vi "Thev-Plot Load Impedances.vi"(2 "State":T1={"next"=-1, "ER10X"=refnum, "phase"=enum."Optimize", "progress"=[], "folder"=path "", "log"="", "history"={"L"=[], "F"=[]}, "optim"={"MSE"=0.0, "Niter"=0, "Linit"=[], "Lfinal"=[]}}, 5 "Mag graph":refnum<vi>, 7 "Phase graph":refnum<vi>, 11 "error in (no error)":errorcluster) -> (15 "error out":errorcluster)   [LabVIEW 2015]
doc: "This helper VI loads calibration data from a file, and plots the magnitude and phase on graphs whose references are inputs to the VI. Handles the logic of overplotting data, selecting the colors and linestyles, and inserting the filename into the legend.\n\nKEH 9/10/09"
uses:
  Typedefs/Thev-State.ctl
  D:/Experiment VIs/Misc VIs/Equipment Control/ER10X/ER10XConnect.NET.dll
  Misc VIs/Equipment Control/ER10X/ER10XConnect.NET.dll
  Typedefs/Thev-Procedure Phase.ctl
  Typedefs/Thev-Progress Table Element.ctl
  Typedefs/Thev-Optimization Result.ctl
  Utility VIs/Math VIs/Z to dB, degrees (1D).vi
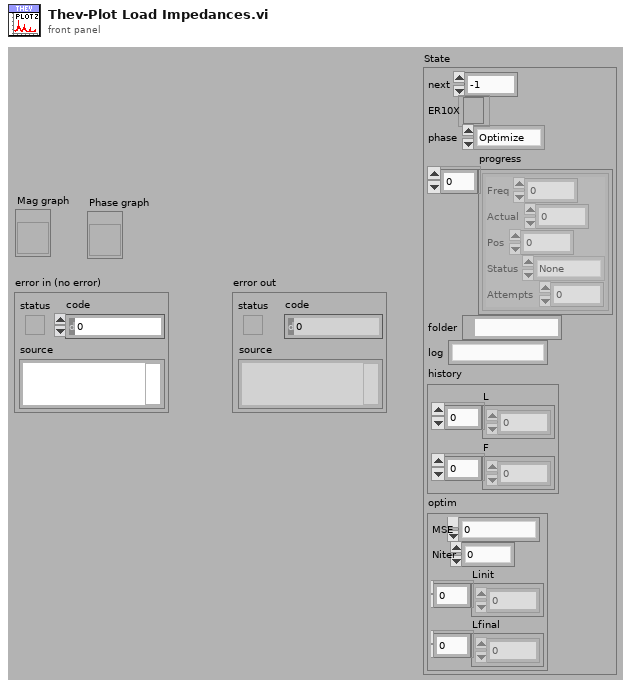
[diagram p1: front panel]
types:
  T1 = typedef "Thev-State.ctl" = cluster{"next":i32, "ER10X":refnum<k24>, "phase":T2, "progress":T3[], "folder":path, "log":string, "history":cluster{"L":dbl[], "F":dbl[]}, "optim":T4}
  T2 = typedef "Thev-Procedure Phase.ctl" = enum16{"Optimize", "Measure", "Compute", "Finished"}
  T3 = typedef "Thev-Progress Table Element.ctl" = cluster{"Freq":dbl, "Actual":dbl, "Pos":dbl, "Status":enum16{"None", "Measuring", "Finished"}, "Attempts":i32}
  T4 = typedef "Thev-Optimization Result.ctl" = cluster{"MSE":dbl, "Niter":i32, "Linit":dbl[], "Lfinal":dbl[]}
  T5 = enum16{"User", "Prism", "Kelly", "Dark2", "Sequential", "Hue"}
  T6 = cluster{"Frequency (Hz)":dbl[], "Magnitude (dB)":dbl[]}
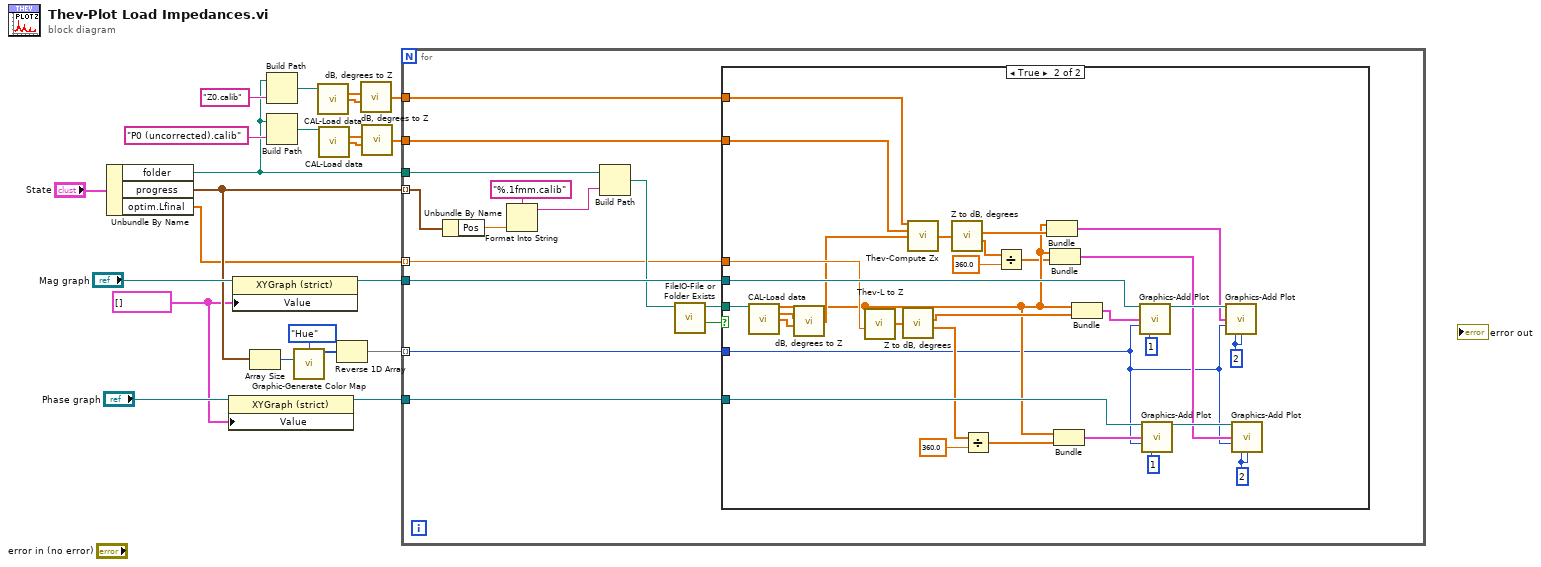
[diagram p0: block diagram]
diagram:
  w13 = cluster{"PTC Mag":dbl[], "PTC Phase":dbl[]}[] [] ("Value")
  n1 = Unbundle By Name("State") -> ("folder"=w9:path, "progress"=w18:T3[], "optim.Lfinal"=w12:dbl[])
  n2 = property class="XYGraph (strict)"(reference="Phase graph", "Value"=w13) -> (reference out=w14:refnum<vi>)  [unwired: 1 in, 1 out]
  n3 = property class="XYGraph (strict)"(reference="Mag graph", "Value"=w13) -> (reference out=w16:refnum<vi>)  [unwired: 1 in, 1 out]
  n4 = Array Size(array=w18) -> (size(s)=w19:i32)
  n5 = Build Path(base path=w9, name or relative path="Z0.calib") -> (appended path=w8:path)
  n6 = Build Path(base path=w9, name or relative path="P0 (uncorrected).calib") -> (appended path=w2:path)
  n7 = call "Graphic-Generate Color Map.vi"("Map"=T5."Hue", "Size"=w19) -> ("Colors"=w20:u32[])  [unwired: 13 in]
  n8 = call "CAL-Load data.vi"("user path"=w8) -> ("Mag"=w7:dbl[], "Phase"=w6:dbl[])  [unwired: 7 in, 6 out]
  n9 = call "CAL-Load data.vi"("user path"=w2) -> ("Mag"=w4:dbl[], "Phase"=w3:dbl[])  [unwired: 7 in, 6 out]
  n10 = Reverse 1D Array(array=w20) -> (reversed array=w17:u32[])
  n11 = call "dB, degrees to Z.vi"("Magnitude (dB)"=w7, "Phase (degrees)"=w6) -> ("Z"=w5:cdb[])  [unwired: 5 in]
  n12 = call "dB, degrees to Z.vi"("Magnitude (dB)"=w4, "Phase (degrees)"=w3) -> ("Z"=w1:cdb[])  [unwired: 5 in]
  n13 = for {
    tunnel: w16 -> [w37]
    tunnel: w9 -> [w32]
    tunnel: w18 -> [w36] mode=indexing
    tunnel: w17 -> [w31] mode=indexing
    tunnel: w14 -> [w27]
    tunnel: w12 -> [w26] mode=indexing
    tunnel: w5 -> [w25]
    tunnel: w1 -> [w24]
    n14 = Unbundle By Name(w36) -> ("Pos"=w34:dbl)
    n15 = Format Into String(format string="%.1fmm.calib", w34) -> (resulting string=w33:string)  [unwired: 2 in, 1 out]
    n16 = Build Path(base path=w32, name or relative path=w33) -> (appended path=w30:path)
    n17 = call "FileIO-File or Folder Exists.vi"("path"=w30) -> ("Exists?"=w28:bool, "dup path"=w29:path)  [unwired: 7 in, 2 out]
    n18 = case shown="True" w28 {
      tunnel: w37 -> [_ w68]
      tunnel: w31 -> [_ w38]
      tunnel: w29 -> [_ w65]
      tunnel: w27 -> [_ w61]
      tunnel: w26 -> [_ w58]
      tunnel: w25 -> [_ w53]
      tunnel: w24 -> [_ w52]
      frame False {
      }
      frame True {
        w45 = u8 2 ("Plot.Line Width")
        w46 = u8 2 ("Plot.Line Width")
        n19 = call "CAL-Load data.vi"("user path"=w65) -> ("Frequency (Hz)"=w41:dbl[], "Mag"=w60:dbl[], "Phase"=w59:dbl[])  [unwired: 7 in, 5 out]
        n20 = call "dB, degrees to Z.vi"("Magnitude (dB)"=w60, "Phase (degrees)"=w59) -> ("Z"=w51:cdb[])  [unwired: 5 in]
        n21 = call "Thev-L to Z.vi"("L (mm)"=w58, "Frequency (Hz)"=w41) -> ("Zx"=w57:cdb[])  [unwired: 2 in]
        n22 = call-poly "Z to dB, degrees.vi"("Z"=w57) -> ("Magnitude (dB)"=w56:dbl[], "Phase (degrees)"=w55:dbl[])  [unwired: 5 in]
        n23 = call "Thev-Compute Zx.vi"("Zs"=w53, "Ps"=w52, "Px"=w51) -> ("Zx"=w49:cdb[])  [unwired: 12 in]
        n24 = call-poly "Z to dB, degrees.vi"("Z"=w49) -> ("Magnitude (dB)"=w48:dbl[], "Phase (degrees)"=w43:dbl[])  [unwired: 5 in]
        n25 = Divide(x=w55, y=360.0) -> (x/y=w54:dbl[])
        n26 = Divide(x=w43, y=360.0) -> (x/y=w40:dbl[])
        n27 = Bundle("Frequency (Hz)"=w41, "Magnitude (dB)"=w48) -> (w47:T6)  [unwired: 1 in]
        n28 = Bundle("Frequency (Hz)"=w41, w40) -> (w39:cluster{"Frequency (Hz)":dbl[], dbl[]})  [unwired: 1 in]
        n29 = Bundle("Frequency (Hz)"=w41, w54) -> (w62:cluster{"Frequency (Hz)":dbl[], dbl[]})  [unwired: 1 in]
        n30 = Bundle("Frequency (Hz)"=w41, "Magnitude (dB)"=w56) -> (w67:T6)  [unwired: 1 in]
        n31 = call "Graphics-Add Plot.vi"("XYGraph in"=w68, "XY Data"=w67, "Color"=w38, "Plot.Line Width"=u8 1) -> ("XYGraph out"=w50:refnum<vi>)  [unwired: 10 in, 1 out]
        n32 = call "Graphics-Add Plot.vi"("XYGraph in"=w61, "XY Data"=w62, "Color"=w38, "Plot.Line Width"=u8 1) -> ("XYGraph out"=w44:refnum<vi>)  [unwired: 10 in, 1 out]
        n33 = call "Graphics-Add Plot.vi"("XYGraph in"=w50, "XY Data"=w47, "Color"=w38, "Plot.Line Width"=w46, "Plot.Line Style"=w46) -> ()  [unwired: 9 in, 2 out]
        n34 = call "Graphics-Add Plot.vi"("XYGraph in"=w44, "XY Data"=w39, "Color"=w38, "Plot.Line Width"=w45, "Plot.Line Style"=w45) -> ()  [unwired: 9 in, 2 out]
      }
    }
  }
